vi "draw 2.vi"() -> ()   [LabVIEW 2009]
uses:
  <vilib>/Utility/miscctls.llb/LVPoint32TypeDef.ctl
  mouse state.ctl
  <vilib>/Utility/cursorutil.llb/Set Cursor (Icon Pict).vi
panel:
  in  "player controls":cluster{"play/pause":bool, "volume":i16}={"play/pause"=TRUE, "volume"=15573} {"volume" scale=0.0..32767.0}
  in  "update sound":bool
  in  "clear waveform":bool
  out "Coords":T1
  out "event":string
  in  "STOP":bool
  out "waveform":u8[](array[slide])=[0, 0, 0, 0, 0, 0, 0, 0, 0, 0, 0, 0, 0, 0, 0, 0, 0, 0, 0, 0, 0, 0, 0, 0, 0, 0, 0, 0, 0, 132, 0, 0, 0, 0, 0, 0, 0, 0, 0, 0, 0, 0, 0, 0, 0, 0, 0, 0, 0, 0, 0, 0, 0, 0, 0, 0, 0, 0, 0, 0, 0, 0, 0, 0, 0, 0, 0, 0, 0, 0, 135, 0, 0, 0, 128, 0, 0, 0, 0, 0, 0, 0, 0, 0, 0, 0, 0, 0, 0, 0, 0, 0, 0, 0, 0, 0, 0, 0, 0, 0, 0, 0, 0, 0, 0, 0, 0, 0, 0, 0, 0, 0, 0, 0, 0, 0, 0, 0, 0, 0, 0, 0, 0, 0, 0, 0, 0, 0, 0, 0, 0, 127, 0, 0, 0, 0, 0, 0, 0, 0, 0, 0, 0, 0, 0, 0, 0, 0, 0, 0, 0, 0, 0, 0, 0, 0, 0, 0, 0, 0, 0, 0, 0, 0, 0, 167, 0, 0, 0, 0, 0, 0, 0, 0, 0, 0, 0, 0, 0, 0, 0, 0, 0, 0, 0, 0, 0, 0, 0, 0, 0, 0, 0, 0, 0] scale=0.0..255.0
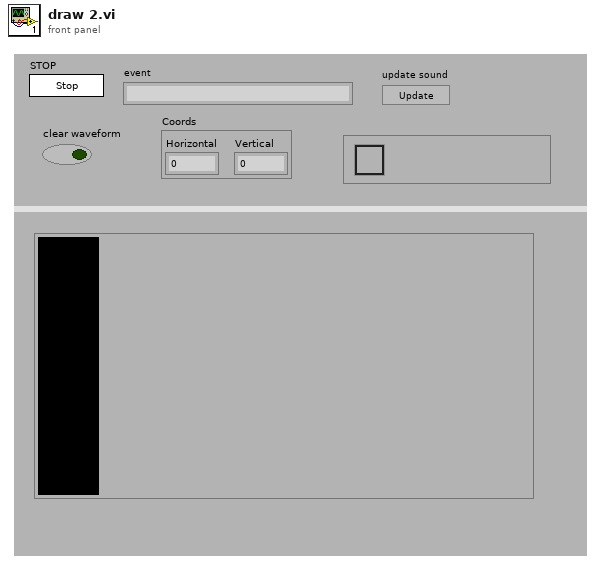
[diagram p1: front panel]
types:
  T1 = typedef "LVPoint32TypeDef.ctl" = cluster{"Horizontal":i32, "Vertical":i32}
  T2 = typedef "mouse state.ctl" = enum16{"ignore", "first", "continue"}
  T3 = enum8{"none", "end", "start", "pause", "update", "volume"}
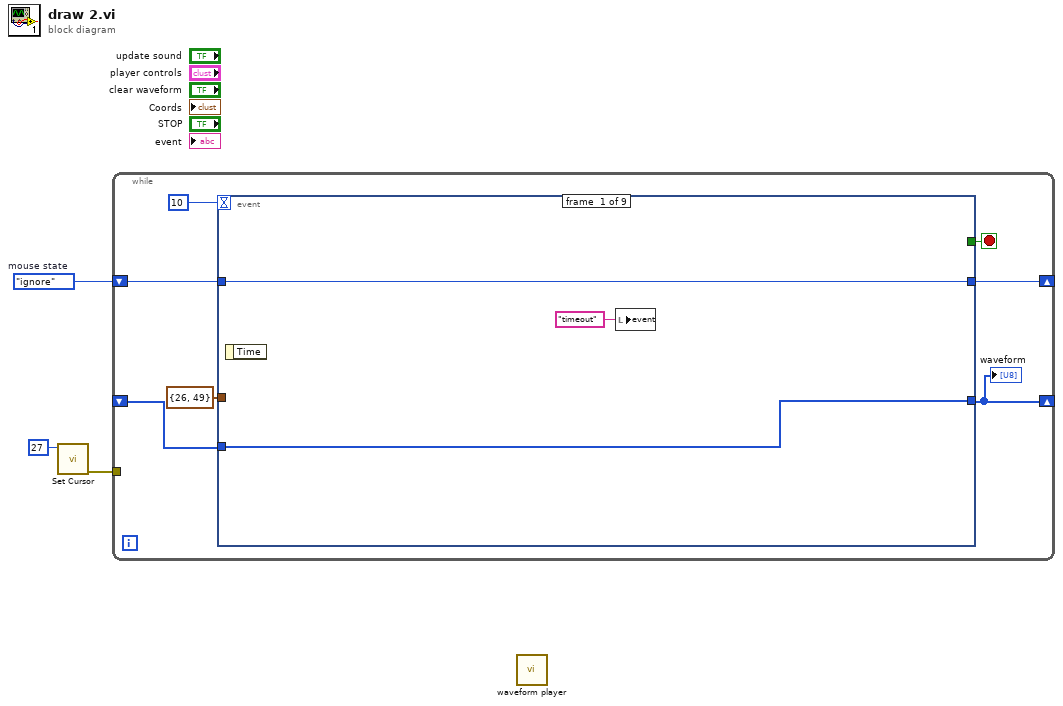
[diagram p0: block diagram]
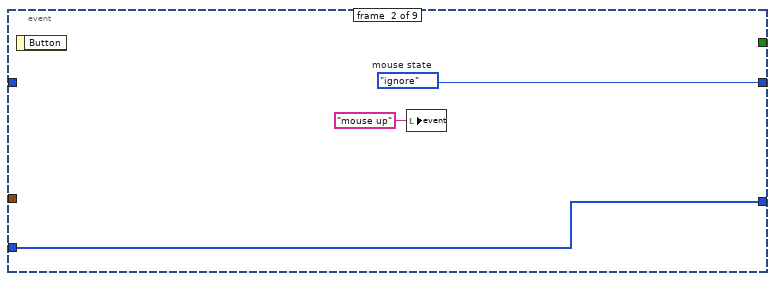
[diagram p2: hidden frame]
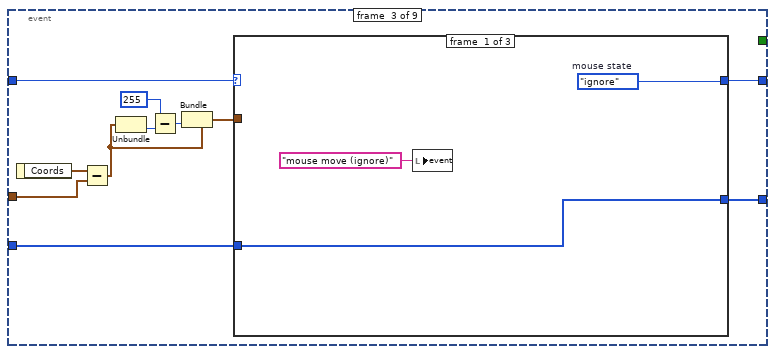
[diagram p3: hidden frame]
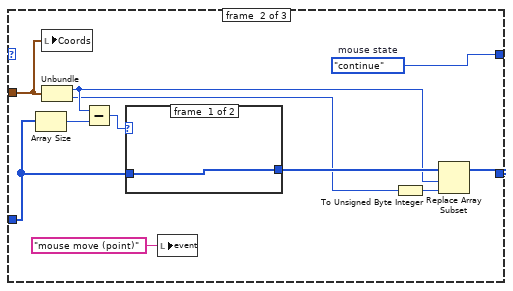
[diagram p4: hidden frame]
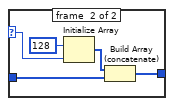
[diagram p5: hidden frame]
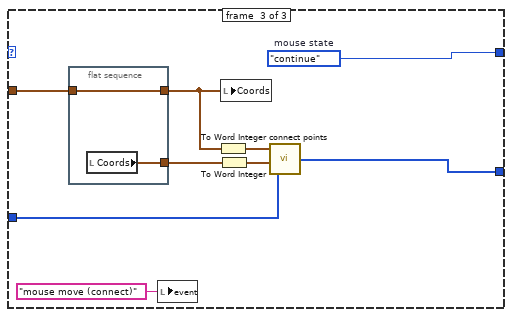
[diagram p6: hidden frame]
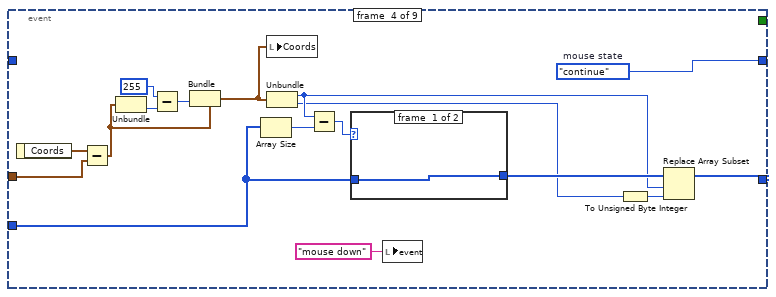
[diagram p7: hidden frame]
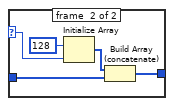
[diagram p8: hidden frame]
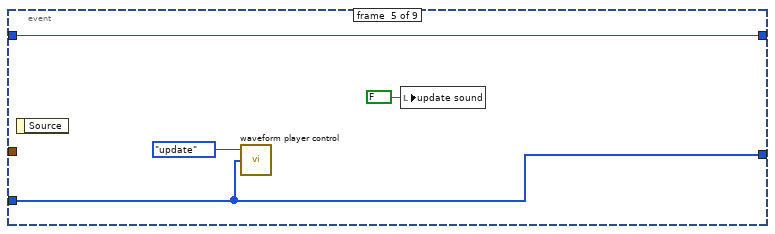
[diagram p9: hidden frame]
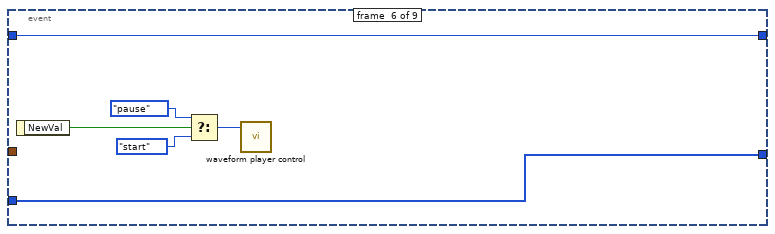
[diagram p10: hidden frame]
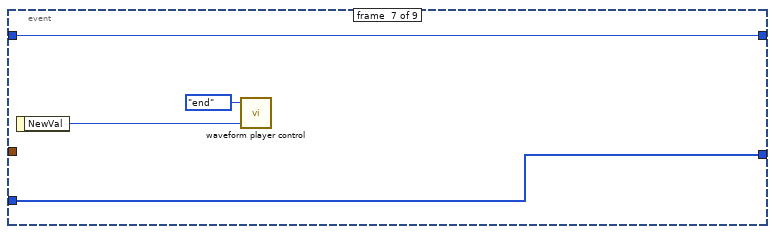
[diagram p11: hidden frame]
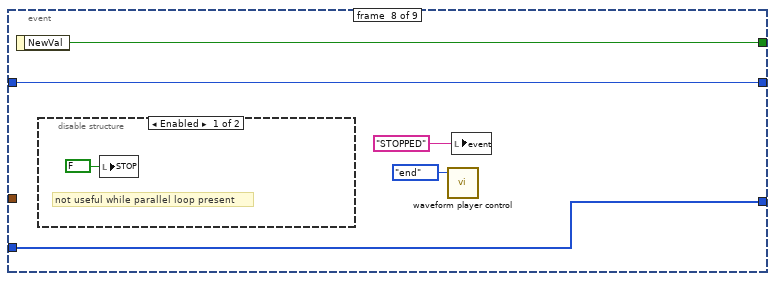
[diagram p12: hidden frame]
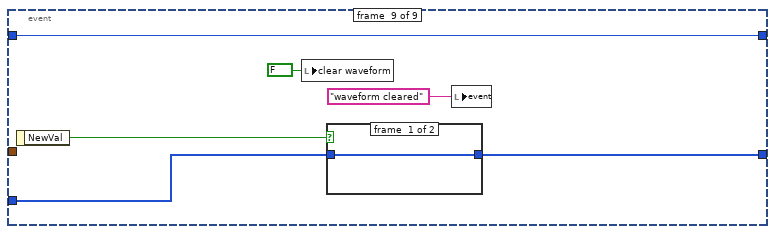
[diagram p14: hidden frame]
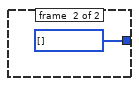
[diagram p15: hidden frame]
diagram:
  w3 = mouse_state."ignore"  # mouse state
  n1 = call-poly <vilib>:"Set Cursor.vi"("icon"=u16 27) -> ("error out"=w1:errorcluster)  [unwired: 9 in, 1 out]
  n2 = while {
    shift-right: [w8] -> _
    shift-left: w3 -> [w9]
    shift-right: [w6] -> _
    shift-left: _ -> [w5]
    tunnel: w1 -> [_]
    stop <- w10 stop-if-true
    n3 = event shown="[7] \"STOP\": Value Change" {
      selector: _ -> [_ _ _ _ _ _ _ _ _]
      dyn-events: _ -> [_ _ _ _ _ _ _ _ _]
      timeout: 10 -> [_ _ _ _ _ _ _ _ _]
      tunnel: [_ _ _ _ _ _ _ w100 _] -> w10
      tunnel: w9 -> [w12 _ w27 _ w84 w90 w94 w98 w106]
      tunnel: [w12 w15 w26 w75 w84 w90 w94 w98 w106] -> w8
      tunnel: w5 -> [w11 w14 w25 w74 w85 w91 w95 w97 w102]
      tunnel: [w11 w14 w24 w73 w85 w91 w95 w97 w105] -> w6
      tunnel: T1 {"Horizontal"=26, "Vertical"=49} ("y") -> [_ _ w17 w59 _ _ _ _ _]
      event #0 {
        n4 = event-data() -> ()  [unwired: 1 in, 1 out]
        n5 = local write "event"("timeout" ("event")) -> ()
      }
      event #1 {
        w15 = mouse_state."ignore"  # mouse state
        n6 = event-data() -> ()  [unwired: 1 in, 1 out]
        n7 = local write "event"("mouse up" ("event")) -> ()
      }
      event #2 {
        n8 = event-data() -> ("Coords"=w23:T1)  [unwired: 1 in]
        n9 = Subtract(x=w23, y=w17) -> (x-y=w22:T1)
        n10 = Unbundle(w22) -> ("Vertical"=w18:i32)  [unwired: 1 out]
        n11 = Subtract(x=255 ("Horizontal"), y=w18) -> (x-y=w19:i32)
        n12 = Bundle(cluster=w22, "Vertical"=w19) -> (w20:T1)  [unwired: 1 in]
        n13 = case shown="\"continue\"" w27 {
          tunnel: w20 -> [_ w33 w52]
          tunnel: [w29 w32 w50] -> w26
          tunnel: w25 -> [w28 w35 w53]
          tunnel: [w28 w34 w51] -> w24
          frame #0 {
            w29 = mouse_state."ignore"  # mouse state
            n14 = local write "event"("mouse move (ignore)" ("event")) -> ()
          }
          frame #1 {
            w32 = mouse_state."continue"  # mouse state
            n15 = Array Size(array=w35) -> (size(s)=w41:i32)
            n16 = local write "Coords"(w33) -> ()
            n17 = Unbundle(w33) -> ("Horizontal"=w38:i32, "Vertical"=w31:i32)
            n18 = Subtract(x=w38, y=w41) -> (x-y=w40:i32)
            n19 = case shown="1.." w40 {
              selector: w40 -> [_ w47]
              tunnel: w35 -> [w42 w45]
              tunnel: [w42 w43] -> w39
              frame #0 {
              }
              frame #1 {
                n20 = Initialize Array(u8 128 ("unsigned 8bit integer"), w47) -> (w44:u8[])
                n21 = Build Array (concatenate)(w44, w45) -> (w43:u8[])
              }
            }
            n22 = local write "event"("mouse move (point)" ("event")) -> ()
            n23 = To Unsigned Byte Integer(number=w31) -> (unsigned 8bit integer=w36:u8)
            n24 = Replace Array Subset(array=w39, new element=w36, index=w38) -> (w34:u8[])
          }
          frame #2 {
            w50 = mouse_state."continue"  # mouse state
            n25 = flat-sequence {
              tunnel: [w57] -> w55
              tunnel: [w58] -> w54
              tunnel: w52 -> [w57]
              frame #0 {
                n26 = local read "Coords"() -> (w58:T1)
              }
            }
            n27 = local write "event"("mouse move (connect)" ("event")) -> ()
            n28 = To Word Integer(number=w55) -> (16bit integer=w49:cluster{"Horizontal":i16, "Vertical":i16})
            n29 = To Word Integer(number=w54) -> (16bit integer=w48:cluster{"Horizontal":i16, "Vertical":i16})
            n30 = local write "Coords"(w55) -> ()
            n31 = call "connect points.vi"("waveform in"=w53, "Coords prev"=w48, "Coords new"=w49) -> ("waveform out"=w51:u8[])
          }
        }
      }
      event #3 {
        w75 = mouse_state."continue"  # mouse state
        n32 = event-data() -> ("Coords"=w72:T1)  [unwired: 1 in]
        n33 = Subtract(x=w72, y=w59) -> (x-y=w71:T1)
        n34 = Unbundle(w71) -> ("Vertical"=w62:i32)  [unwired: 1 out]
        n35 = Subtract(x=255 ("Horizontal"), y=w62) -> (x-y=w60:i32)
        n36 = Bundle(cluster=w71, "Vertical"=w60) -> (w70:T1)  [unwired: 1 in]
        n37 = Array Size(array=w74) -> (size(s)=w69:i32)
        n38 = local write "Coords"(w70) -> ()
        n39 = Unbundle(w70) -> ("Horizontal"=w66:i32, "Vertical"=w63:i32)
        n40 = Subtract(x=w66, y=w69) -> (x-y=w68:i32)
        n41 = case shown="1.." w68 {
          selector: w68 -> [_ w81]
          tunnel: w74 -> [w76 w79]
          tunnel: [w76 w77] -> w67
          frame #0 {
          }
          frame #1 {
            n42 = Initialize Array(u8 128 ("unsigned 8bit integer"), w81) -> (w78:u8[])
            n43 = Build Array (concatenate)(w78, w79) -> (w77:u8[])
          }
        }
        n44 = local write "event"("mouse down" ("event")) -> ()
        n45 = To Unsigned Byte Integer(number=w63) -> (unsigned 8bit integer=w64:u8)
        n46 = Replace Array Subset(array=w67, new element=w64, index=w66) -> (w73:u8[])
      }
      event #4 {
        n47 = event-data() -> ()  [unwired: 1 in, 1 out]
        n48 = call "waveform player control.vi"("type"=T3."update", "waveform"=w85) -> ()  [unwired: 4 in]
        n49 = local write "update sound"(FALSE ("update sound")) -> ()
      }
      event #5 {
        n50 = event-data() -> ("NewVal"=w89:bool)  [unwired: 1 in]
        n51 = Select(t=T3."pause" ("type"), s=w89, f=T3."start" ("type")) -> (s? t:f=w86:T3)
        n52 = call "waveform player control.vi"("type"=w86) -> ()  [unwired: 5 in]
      }
      event #6 {
        n53 = event-data() -> ("NewVal"=w93:i16)  [unwired: 1 in]
        n54 = call "waveform player control.vi"("type"=T3."end", "volume"=w93) -> ()  [unwired: 4 in]
      }
      event #7 {
        n55 = event-data() -> ("NewVal"=w100:bool)  [unwired: 1 in]
        n56 = disable-structure shown="Enabled" {
          frame #0 {
            # "not useful while parallel loop present"
            n57 = local write "STOP"(FALSE ("STOP")) -> ()
          }
          frame #1 {
          }
        }
        n58 = call "waveform player control.vi"("type"=T3."end") -> ()  [unwired: 5 in]
        n59 = local write "event"("STOPPED" ("event")) -> ()
      }
      event #8 {
        n60 = event-data() -> ("NewVal"=w103:bool)  [unwired: 1 in]
        n61 = local write "clear waveform"(FALSE ("clear waveform")) -> ()
        n62 = case shown="False" w103 {
          tunnel: [w108 u8[] [] ("waveform")] -> w105
          tunnel: w102 -> [w108 _]
          frame #0 {
          }
          frame #1 {
          }
        }
        n63 = local write "event"("waveform cleared" ("event")) -> ()
      }
    }
    "waveform" <- w6
  }
  n64 = call "waveform player.vi"() -> ()  [unwired: 2 in]
